vi "VScaleInfoAcq.vi"(0 "Instrument ID":u32, 2 "Channel (1)":i32=1, 3 "error in (no error)":errorcluster) -> (6 "vGain scalar":dbl, 7 "vGain (dB)":dbl, 9 "Total Gain (dB)":dbl, 10 "Voltage Scale":T1)   [LabVIEW 2022 SP3]
uses:
  <instrlib>/Acqiris Dx/Acqiris Dx.lvlib
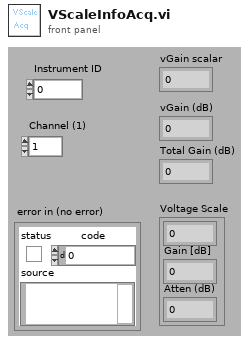
[diagram p1: front panel]
types:
  T1 = cluster{sgl, "Gain [dB]  ":sgl, "Atten (dB)":sgl}
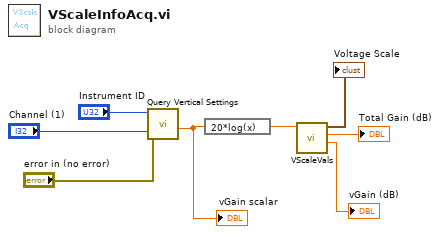
[diagram p0: block diagram]
diagram:
  n1 = call <instrlib>:"Query Vertical Settings.vi"("Instrument ID"="Instrument ID", "Channel (1)"="Channel (1)", "error in (no error)"="error in (no error)") -> ("Full Scale"=w4:dbl)  [unwired: 6 out]
  "vGain scalar" <- w4
  n2 = expression code="20*log(x)"(w4) -> (w6:dbl)
  n3 = call "VScaleVals.vi"("Full Scale"=w6) -> ("vGain (dB)"=→"vGain (dB)":dbl, "Total Gain (dB)"=→"Total Gain (dB)":dbl, "Voltage Scale"=→"Voltage Scale":T1)  [unwired: 8 in]
